vi "Trapezoidal Set RPM.vi"(8 "Desired RPM":dbl, 9 "Current RPM":dbl, 11 "Spinning Wheels?":bool) -> (2 "Stage 1 Time":dbl, 3 "RPM":dbl, 5 "Shooter Ready?":bool)   [LabVIEW 2015]
uses:
  Trapezoidal Motion State.ctl
  Common Code/Change Detect Boolean.vi
  Common Code/Change Detect Double.vi
  Robot Code/Robot Global Data.vi
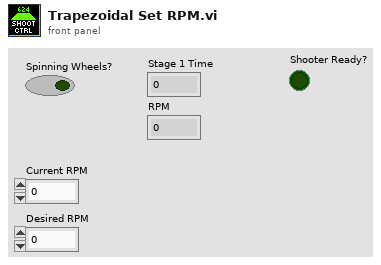
[diagram p1: front panel]
types:
  T1 = typedef "Trapezoidal Motion State.ctl" = enum16{"Accelerate", "Cruise", "Decelerate", "Finish"}
  T2 = typedef "Dashboard Control Data.ctl" = cluster{"Shooter Presets":T3, "Encoder Control":T5, "Steer PID output":cluster{"output high":dbl, "output low":dbl}, " Steer PID gains":cluster{"proportional gain (Kc)":dbl, "integral time (Ti, min)":dbl, "derivative time (Td, min)":dbl}, "Drivetrain Settings":T6, "Vision Packet":T7, "Dashboard Drivetrain Command":T8, "Info/Command Cluster":T10, "Ball Vision Packet":T11, "Intake Presets":T13, "Intake Encoder Control":T15, "Climb Presets":T16, "Ultrasonic Limit":dbl, "Roll Limit":dbl, "Pitch Limit":dbl, "Goal Output Range":cluster{"output high":dbl, "output low":dbl}}
  T3 = typedef "Shooter Presets.ctl" = cluster{"Batter Shot":T4, "Deep Middle Shot":T4, "Manual Shot":T4, "Left Ticks Per Rotation":dbl, "Right Ticks Per Rotation":dbl, "Low Bar Shot":T4, "Shooter RPM Tolerance":dbl, "IIR Filter Power":dbl, "Trigger Power":dbl, "Fire from Load Delay":i32, "Angle Pot M":dbl, "Angle Pot B":dbl, "Shooter Length":dbl, "String Pot Dist":dbl, "Angle PID gains":cluster{"proportional gain (Kc)":dbl, "integral time (Ti, min)":dbl, "derivative time (Td, min)":dbl}, "Angle Motor Output":cluster{"output high":dbl, "output low":dbl}, "Shooter Angle Tolerance":dbl, "Vision Shoot x^2":dbl, "Vision Shoot x":dbl, "Dist from Axis Cam to Pivot":dbl, "High Goal Center Height":dbl, "Feed Forward Max Accel":dbl, "Feed Forward Kv":dbl, "Backwards Trigger":dbl, "Shot Finish Delay (ms)":dbl, "Angle Max Current":dbl, "Angle Current Trip Time":dbl, "Shooter Intake Angle":dbl, "Vision Shoot c":dbl, "Reset?":bool, "Servo Release Delay":dbl, "Servo Idle Angle":i32, "Servo Hold Angle":i32, "Angle Pot x^2":dbl, "Angle Pot x":dbl, "Angle Pot c":dbl, "Ignore Angle?":bool}
  T4 = typedef "Shot Presets.ctl" = cluster{"Left Wheel RPM":dbl, "Right Wheel RPM":dbl, "Angle":dbl}
  T5 = typedef "Encoder Control.ctl" = cluster{"Right Tick Constant":dbl, "Left Tick Constant":dbl, "Reset?":bool, "Y Dist":cluster{"PID gains":cluster{"proportional gain (Kc)":dbl, "integral time (Ti, min)":dbl, "derivative time (Td, min)":dbl}}, "Y Stop Thresh":dbl, "Y Stop Speed":dbl}
  T6 = typedef "Drivetrain Settings.ctl" = cluster{"Gyro Tolerance":dbl, "Throttle Ramp (ms)":dbl, "Angular rate compensation":bool, "Throttle to Rate Scale":dbl, "Rate compensation gain":dbl, "Kv":dbl, "Ka":dbl, "Feed Forward P":dbl, "Feed Forward D":dbl, "Goal Vision PID gains":cluster{"proportional gain (Kc)":dbl, "integral time (Ti, min)":dbl, "derivative time (Td, min)":dbl}, "Goal Detection Window":dbl}
  T7 = typedef "Goal Vision Packet.ctl" = cluster{"Distance":dbl, "Center X":dbl, "Center Y":dbl, "Found Target?":bool}
  T8 = typedef "Dashboard Drivetrain Command.ctl" = cluster{"Drivetrain Vision":T9}
  T9 = typedef "Drivetrain Vision.ctl" = cluster{"Goal Window":dbl, "Ball Window":dbl}
  T10 = typedef "Ball Tracking Command Cluster.ctl" = cluster{"Distance to Ball":dbl, "Desired Angle":dbl, "Command":enum16{"Turn to Ball", "Turn to Angle", "Get Distance"}, "Pixels from Center":dbl}
  T11 = typedef "Ball Vision Packet.ctl" = cluster{"Ball Detected?":bool, "Distance to Ball":dbl, "Desired Angle":dbl, "Pixels from Center":dbl, "Tracking mode":T12}
  T12 = typedef "Tracking Mode.ctl" = enum16{"Turn to Ball", "Turn to Angle"}
  T13 = typedef "Intake Presets.ctl" = cluster{"Intake Speed":dbl, "Outake Speed":dbl, "Low Height":dbl, "Half Height":dbl, "Full Height":dbl, "Angle Speed":dbl, "Fast Angle":dbl, "Encoder Scale":dbl, "Load Height":dbl, "Output Range":T14, "Rotation Power Max/Min":dbl, "MaxCurrent":dbl, "Intake Trip Time":dbl, "Idle Height":dbl, "Max Height":dbl, "Reset Encoders?":bool, "PID gains":cluster{"proportional gain (Kc)":dbl, "integral time (Ti, min)":dbl, "derivative time (Td, min)":dbl}}
  T14 = typedef "Drivetrain Output Range.ctl" = cluster{"output high":dbl, "output low":dbl}
  T15 = typedef "IntakeEcoderControl.ctl" = cluster{"Arm Tick Constant":dbl, "Reset?":bool, "Y Dist":cluster{"PID gains":cluster{"proportional gain (Kc)":dbl, "integral time (Ti, min)":dbl, "derivative time (Td, min)":dbl}}, "Y Stop Thresh":dbl, "Y Stop Speed":dbl}
  T16 = typedef "Climb Presets.ctl" = cluster{"Pull Power":dbl, "Unpin Power":dbl, "Time to Hold":dbl}
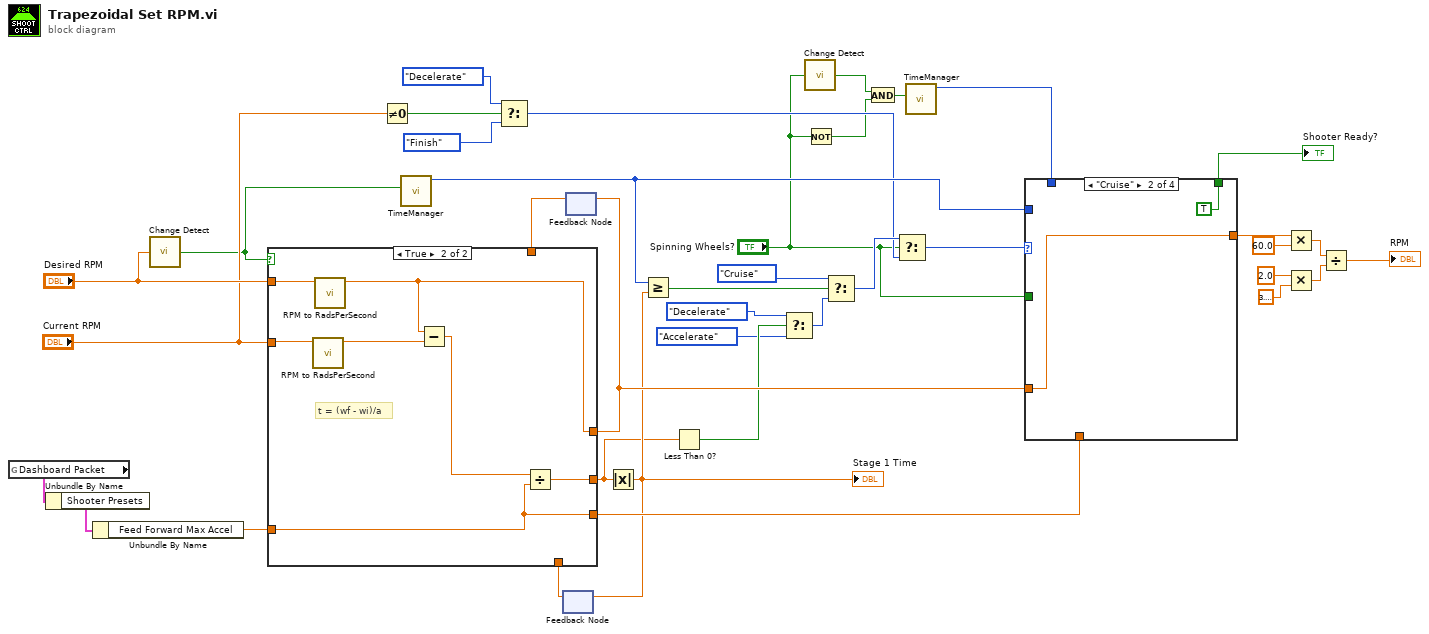
[diagram p0: block diagram]
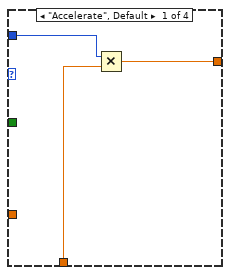
[diagram p2: hidden frame]
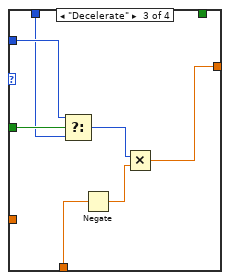
[diagram p3: hidden frame]
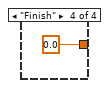
[diagram p4: hidden frame]
diagram:
  n1 = global read "Robot Global Data.vi" "Dashboard Packet"() -> (w20:T2)
  n2 = Unbundle By Name(w20) -> ("Shooter Presets"=w21:T3)
  n3 = Unbundle By Name(w21) -> ("Feed Forward Max Accel"=w19:dbl)
  n4 = call-poly "Change Detect.vi"("In"="Desired RPM") -> ("Changed?"=w1:bool)
  n5 = Not Equal To 0?(x="Current RPM") -> (x != 0?=w11:bool)
  n6 = call "TimeManager.vi"("Reset?"=w1) -> ("Time Since Reset"=w32:u32)  [unwired: 9 in, 1 out]
  n7 = Select(t=Trapezoidal_Motion_State."Decelerate" ("Enum"), s=w11, f=Trapezoidal_Motion_State."Finish" ("Enum")) -> (s? t:f=w8:T1)
  n8 = feedback #1() -> (w37:dbl)  [unwired: 1 in]
  n9 = feedback #2() -> (w23:dbl)  [unwired: 1 in]
  n10 = case shown="True" w1 {
    tunnel: [w41 w48] -> w17
    tunnel: "Current RPM" -> [_ w45]
    tunnel: "Desired RPM" -> [_ w46]
    tunnel: w37 -> [w41 _]
    tunnel: [w39 w47] -> w31
    tunnel: [w40 w42] -> w22
    tunnel: w23 -> [w40 _]
    tunnel: w19 -> [w39 w47]
    frame False {
    }
    frame True {
      # "t = (wf - wi)/a"
      n11 = call "RPM to RadsPerSecond.vi"("Desired RPM"=w45) -> ("Numeric"=w44:dbl)  [unwired: 10 in]
      n12 = call "RPM to RadsPerSecond.vi"("Desired RPM"=w46) -> ("Numeric"=w42:dbl)  [unwired: 10 in]
      n13 = Subtract(x=w42, y=w44) -> (x-y=w43:dbl)
      n14 = Divide(x=w43, y=w47) -> (x/y=w48:dbl)
    }
  }
  n15 = feedback-in #2(w22) -> ()
  n16 = Absolute Value(x=w17) -> (abs(x)=w18:dbl)
  "Stage 1 Time" <- w18
  n17 = feedback-in #1(w18) -> ()
  n18 = Greater Or Equal?(x=w32, y=w18) -> (x >= y?=w36:bool)
  n19 = Less Than 0?(x=w17) -> (x < 0?=w16:bool)
  n20 = Select(t=Trapezoidal_Motion_State."Decelerate" ("Enum"), s=w16, f=Trapezoidal_Motion_State."Accelerate") -> (s? t:f=w13:T1)
  n21 = call-poly "Change Detect.vi"("In"="Spinning Wheels?") -> ("Changed?"=w7:bool)
  n22 = Not(x="Spinning Wheels?") -> (.not. x?=w6:bool)
  n23 = Select(t=Trapezoidal_Motion_State."Cruise" ("Enum"), s=w36, f=w13) -> (s? t:f=w34:T1)
  n24 = And(x=w7, y=w6) -> (x .and. y?=w5:bool)
  n25 = Select(t=w34, s="Spinning Wheels?", f=w8) -> (s? t:f=w33:T1)
  n26 = call "TimeManager.vi"("Reset?"=w5) -> ("Time Since Reset"=w3:u32)  [unwired: 9 in, 1 out]
  n27 = case shown="\"Cruise\"" w33 {
    tunnel: w32 -> [w51 _ w58 _]
    tunnel: w31 -> [w49 _ w60 _]
    tunnel: [w50 w53 w55 0.0] -> w30
    tunnel: w22 -> [_ w53 _ _]
    tunnel: "Spinning Wheels?" -> [_ _ w59 _]
    tunnel: w3 -> [_ _ w54 _]
    tunnel: [_ TRUE _ _] -> w2
    frame "Accelerate", Default {
      n28 = Multiply(x=w51, y=w49) -> (x*y=w50:dbl)
    }
    frame "Cruise" {
    }
    frame "Decelerate" {
      n29 = Select(t=w58, s=w59, f=w54) -> (s? t:f=w57:u32)
      n30 = Negate(x=w60) -> (-x=w56:dbl)
      n31 = Multiply(x=w57, y=w56) -> (x*y=w55:dbl)
    }
    frame "Finish" {
    }
  }
  "Shooter Ready?" <- w2
  n32 = Multiply(x=w30, y=60.0) -> (x*y=w26:dbl)
  n33 = Multiply(x=2.0, y=3.141592653589793) -> (x*y=w25:dbl)
  n34 = Divide(x=w26, y=w25) -> (x/y=→"RPM":dbl)
